vi "Box_Inside_Envelope.vi"(2 "Box to check":T1=[{"Max"=16000.0, "Min"=14000.0}, {"Max"=1000.0, "Min"=-1000.0}, {"Max"=700.0, "Min"=0.0}] {"Min" format="%#.1f"; "Max" format="%#.1f"}, 3 "Envelope":T1=[{"Max"=16000.0, "Min"=14000.0}, {"Max"=1000.0, "Min"=-1000.0}, {"Max"=700.0, "Min"=0.0}] {"Min" format="%#.1f"; "Max" format="%#.1f"}) -> (0 "Error Comments":string, 1 "Box Inside":bool)   [LabVIEW 2010]
uses:
  Box_size.ctl
panel:
  # "X                           Y                          Z"
  # "X                           Y                          Z"
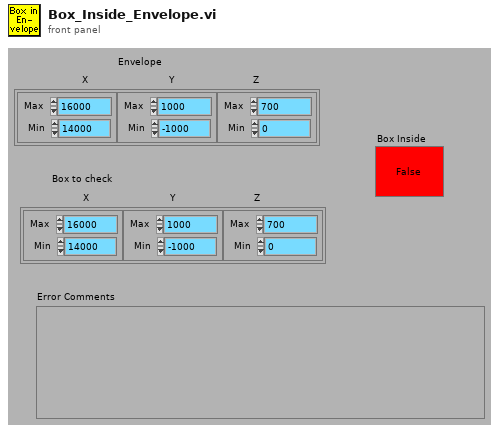
[diagram p1: front panel]
types:
  T1 = typedef "Box_size.ctl" = cluster{"Max":dbl, "Min":dbl}[]
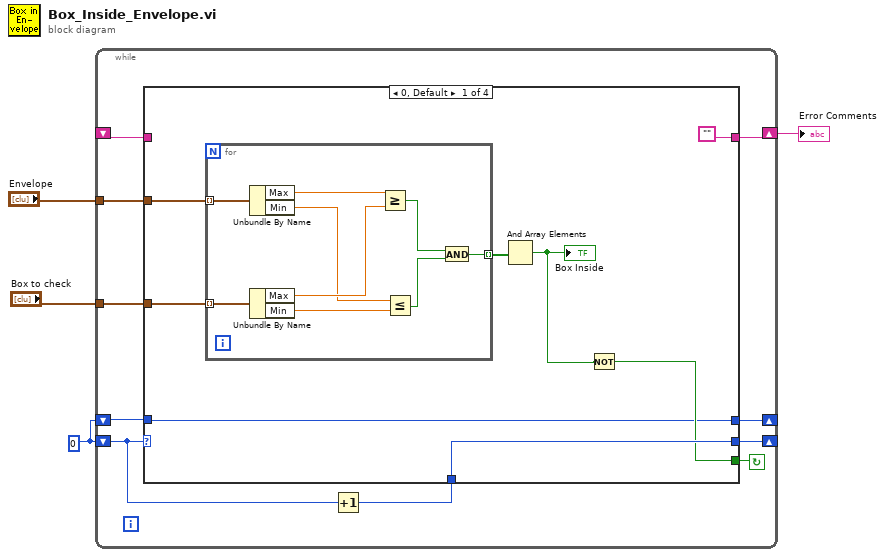
[diagram p0: block diagram]
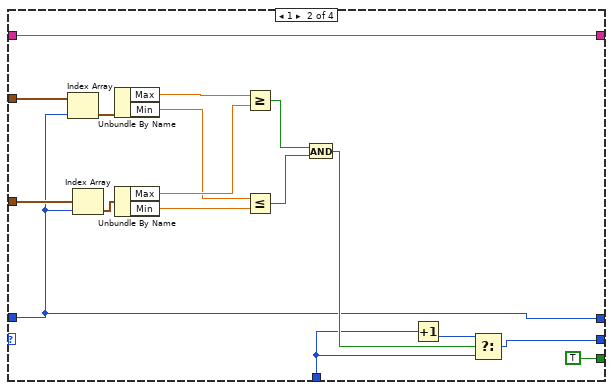
[diagram p2: hidden frame]
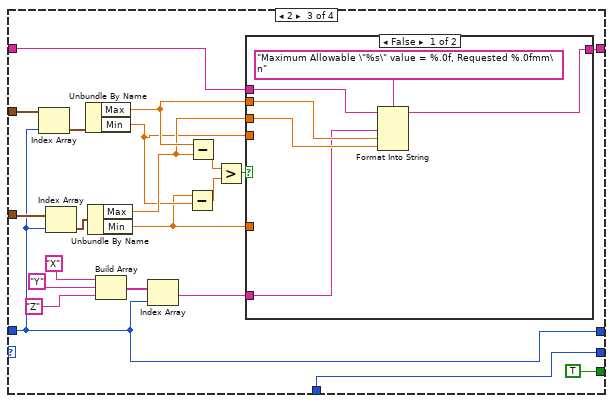
[diagram p3: hidden frame]
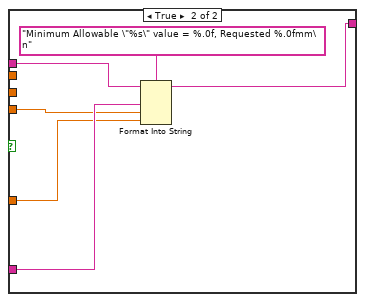
[diagram p4: hidden frame]
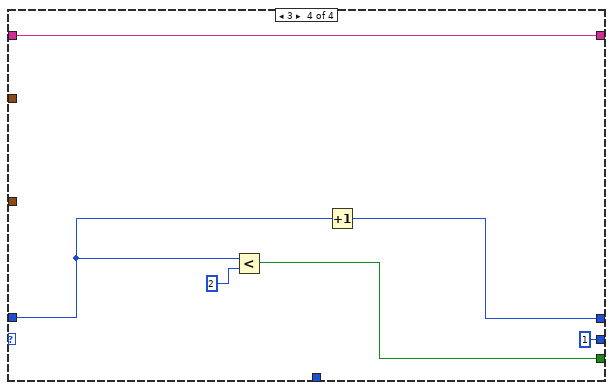
[diagram p5: hidden frame]
diagram:
  w1 = 0
  n1 = while {
    shift-left: w1 -> [w7]
    shift-right: [w6] -> _
    shift-left: _ -> [w5]
    shift-right: [w8] -> w2
    shift-left: w1 -> [w12]
    shift-right: [w10] -> _
    tunnel: "Box to check" -> [w13]
    tunnel: "Envelope" -> [w14]
    stop <- w9 continue-if-true
    n2 = Increment(x=w12) -> (x+1=w11:i32)
    n3 = case shown="0, Default" w12 {
      tunnel: w14 -> [w22 w42 w63 _]
      tunnel: w13 -> [w21 w41 w62 _]
      tunnel: w11 -> [w19 w36 w51 _]
      tunnel: [w19 w35 w51 1] -> w10
      tunnel: [w17 TRUE TRUE w86] -> w9
      tunnel: ["" w32 w54 w82] -> w8
      tunnel: w7 -> [w15 w34 w49 w85]
      tunnel: [w15 w34 w49 w84] -> w6
      tunnel: w5 -> [_ w32 w55 w82]
      frame 0, Default {
        n4 = for {
          tunnel: w22 -> [w31] mode=indexing
          tunnel: w21 -> [w30] mode=indexing
          tunnel: [w23] -> w20 mode=indexing
          n5 = Unbundle By Name(w31) -> ("Max"=w29:dbl, "Min"=w27:dbl)
          n6 = Unbundle By Name(w30) -> ("Max"=w28:dbl, "Min"=w26:dbl)
          n7 = Greater Or Equal?(x=w29, y=w28) -> (x >= y?=w25:bool)
          n8 = Less Or Equal?(x=w27, y=w26) -> (x <= y?=w24:bool)
          n9 = And(x=w25, y=w24) -> (x .and. y?=w23:bool)
        }
        n10 = And Array Elements(Boolean array=w20) -> (logical AND=w18:bool)
        "Box Inside" <- w18
        n11 = Not(x=w18) -> (.not. x?=w17:bool)
      }
      frame 1 {
        n12 = Index Array(array=w42, index=w34) -> (element=w39:cluster{"Max":dbl, "Min":dbl})
        n13 = Index Array(array=w41, index=w34) -> (element=w40:cluster{"Max":dbl, "Min":dbl})
        n14 = Unbundle By Name(w39) -> ("Max"=w48:dbl, "Min"=w45:dbl)
        n15 = Unbundle By Name(w40) -> ("Max"=w47:dbl, "Min"=w46:dbl)
        n16 = Greater Or Equal?(x=w48, y=w47) -> (x >= y?=w44:bool)
        n17 = Less Or Equal?(x=w45, y=w46) -> (x <= y?=w43:bool)
        n18 = And(x=w44, y=w43) -> (x .and. y?=w38:bool)
        n19 = Increment(x=w36) -> (x+1=w37:i32)
        n20 = Select(t=w37, s=w38, f=w36) -> (s? t:f=w35:i32)
      }
      frame 2 {
        n21 = Index Array(array=w63, index=w49) -> (element=w64:cluster{"Max":dbl, "Min":dbl})
        n22 = Index Array(array=w62, index=w49) -> (element=w65:cluster{"Max":dbl, "Min":dbl})
        n23 = Unbundle By Name(w64) -> ("Max"=w58:dbl, "Min"=w53:dbl)
        n24 = Unbundle By Name(w65) -> ("Max"=w57:dbl, "Min"=w52:dbl)
        n25 = Build Array("X", "Y", "Z") -> (w66:string[])
        n26 = Index Array(array=w66, index=w49) -> (element=w56:string)
        n27 = Subtract(x=w52, y=w53) -> (x-y=w61:dbl)
        n28 = Subtract(x=w58, y=w57) -> (x-y=w60:dbl)
        n29 = Greater?(x=w60, y=w61) -> (0:w59:bool)
        n30 = case shown="False" w59 {
          tunnel: w58 -> [w75 _]
          tunnel: w57 -> [w74 _]
          tunnel: w56 -> [w72 w81]
          tunnel: w55 -> [w71 w80]
          tunnel: [w70 w79] -> w54
          tunnel: w53 -> [_ w78]
          tunnel: w52 -> [_ w77]
          frame False {
            n31 = Format Into String(format string="Maximum Allowable \"%s\" value = %.0f, Requested %.0fmm\n" ("Format String"), initial string=w71, w72, w75, w74) -> (resulting string=w70:string)  [unwired: 1 in, 1 out]
          }
          frame True {
            n32 = Format Into String(format string="Minimum Allowable \"%s\" value = %.0f, Requested %.0fmm\n" ("Format String"), initial string=w80, w81, w78, w77) -> (resulting string=w79:string)  [unwired: 1 in, 1 out]
          }
        }
      }
      frame 3 {
        n33 = Less?(x=w85, y=2) -> (x < y?=w86:bool)
        n34 = Increment(x=w85) -> (x+1=w84:i32)
      }
    }
  }
  "Error Comments" <- w2
